vi "AddTransaction.vi"(8 "error in (no error)":errorcluster, 10 "Transaction.lvclass":refnum<class "Transaction.lvclass">, 11 "TransactionList in":refnum<class "TransactionList.lvclass">) -> (0 "error out":errorcluster, 3 "TransactionList out":refnum<class "TransactionList.lvclass">)   [LabVIEW 2018, in "TransactionList.lvclass"]
uses:
  TransactionList.lvclass
  Transaction/Transaction.lvclass
  TransactionList.lvclass/TransactionList.ctl
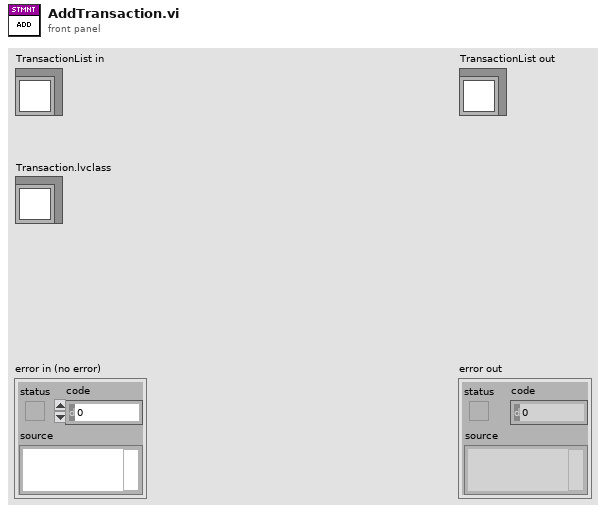
[diagram p1: front panel]
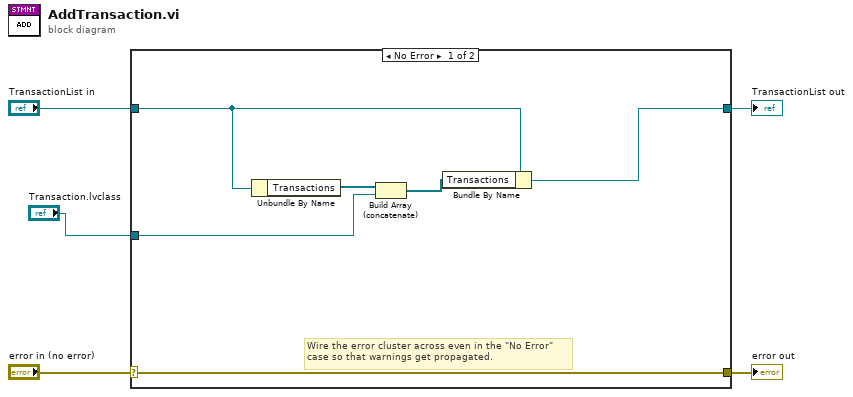
[diagram p0: block diagram]
diagram:
  n1 = case shown="No Error" "error in (no error)" {
    selector: "error in (no error)" -> [w11 w13]
    tunnel: [w11 w13] -> w4
    tunnel: [w10 w12] -> w2
    tunnel: "TransactionList in" -> [w9 w12]
    tunnel: "Transaction.lvclass" -> [w6 _]
    frame No Error {
      # "Wire the error cluster across even in the \"No Error\"\ncase so that warnings get propagated."
      n2 = Unbundle By Name(w9) -> ("Transactions"=w8:refnum<class "Transaction.lvclass">[])
      n3 = Build Array (concatenate)(w8, w6) -> (w7:refnum<class "Transaction.lvclass">[])
      n4 = Bundle By Name(cluster=w9, "Transactions"=w7) -> (w10:refnum<class "TransactionList.lvclass">)
    }
    frame Error {
    }
  }
  "error out" <- w4
  "TransactionList out" <- w2
